vi "Delay.vi"(0 "Delay Time (s)":dbl=1.0 caption="延迟时间(s)", 2 "error in (no error)":errorcluster caption="错误输入（无错误）") -> (16 "error out":errorcluster caption="错误输出")   [LabVIEW 2015, in "UARTCOM.lvlib"]
uses:
  UARTCOM.lvlib
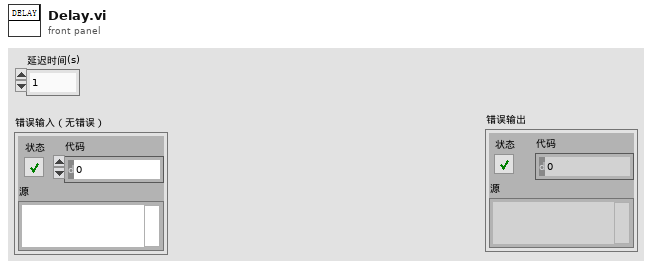
[diagram p1: front panel]
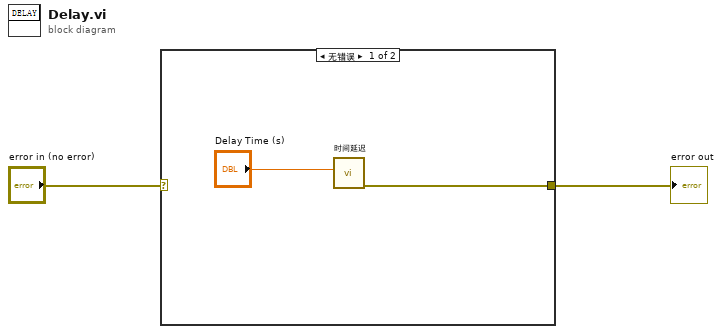
[diagram p0: block diagram]
diagram:
  n1 = case shown="无错误" "error in (no error)" {
    selector: "error in (no error)" -> [_ w5]
    tunnel: [w4 w5] -> w1
    frame No Error {
      n2 = call "时间延迟"("Delay Time (s)"="Delay Time (s)") -> ("error out"=w4:errorcluster)  [unwired: 10 in]
    }
    frame Error {
    }
  }
  "error out" <- w1
